vi "publicFunctionInBase.vi"(11 "String In":string) -> (3 "String Out":string)   [LabVIEW 2013, in "Base.lvlib"]
uses:
  Base.lvlib
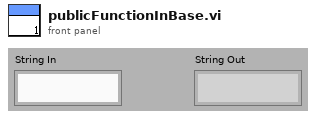
[diagram p1: front panel]
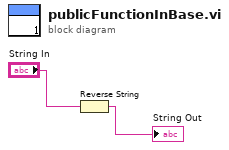
[diagram p0: block diagram]
diagram:
  n1 = Reverse String(1:"String In") -> (0:→"String Out":string)
